vi "Write_Ch_data_file.vi"(4 "Append last row only":bool, 5 "Header string":string, 7 "exists?":bool, 8 "Write offset fr file end":i32, 9 "Channel Values":string[][](array[string]), 10 "Channel names":string[](array[string]), 11 "Filename":path) -> ()   [LabVIEW 2015]
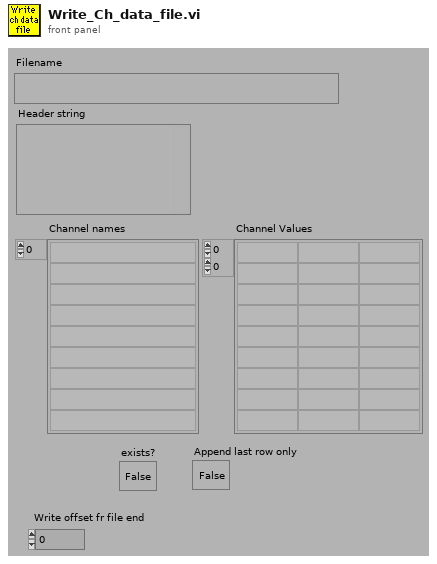
[diagram p1: front panel]
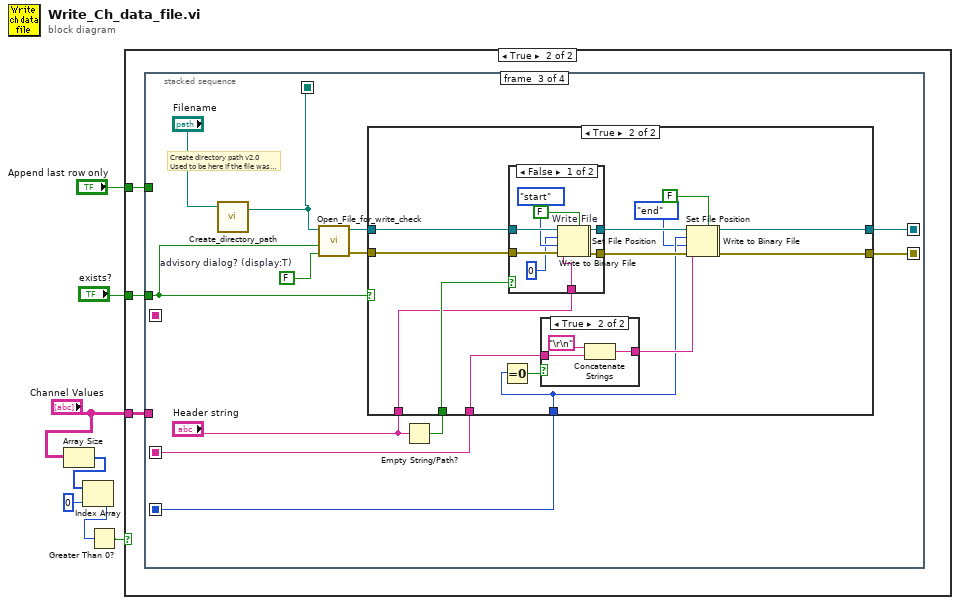
[diagram p0: block diagram]
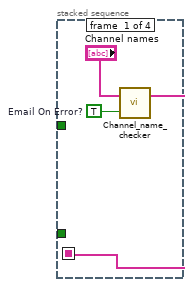
[diagram p3: hidden frame]
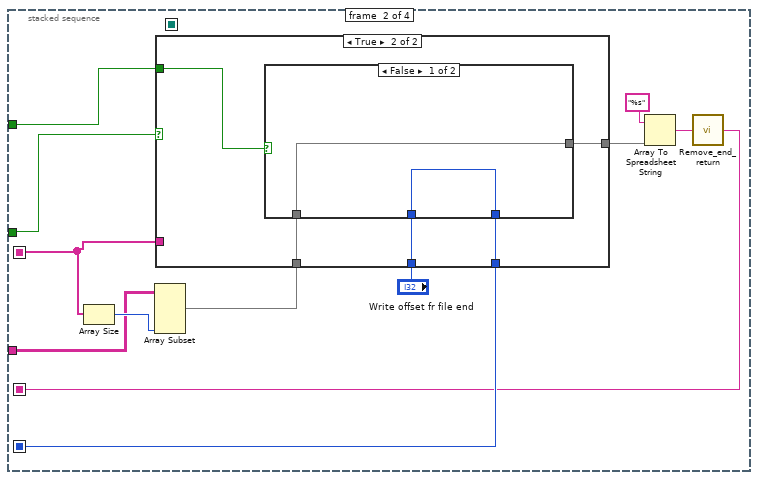
[diagram p4: hidden frame]
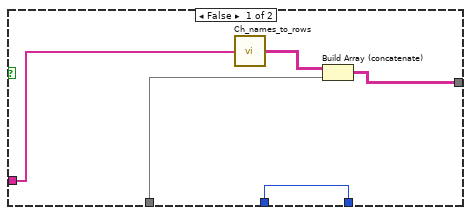
[diagram p5: hidden frame]
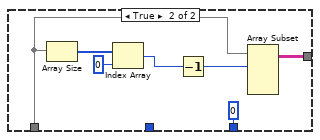
[diagram p6: hidden frame]
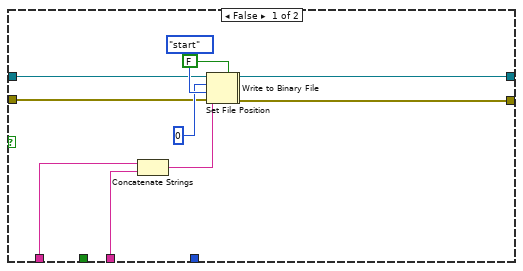
[diagram p7: hidden frame]
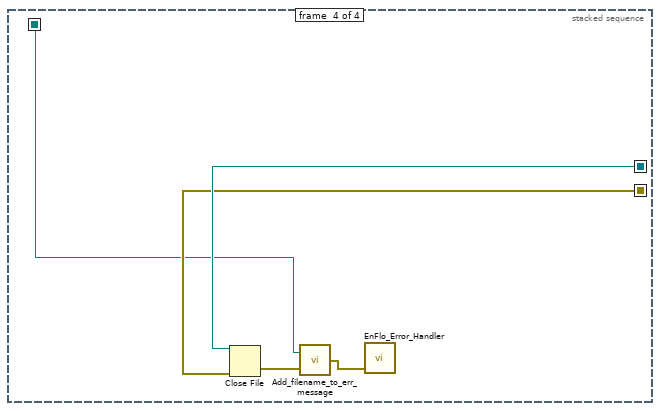
[diagram p10: hidden frame]
diagram:
  n1 = Array Size(array="Channel Values") -> (size(s)=w3:i32[])
  n2 = Index Array(array=w3, index=0 ("Index")) -> (element=w2:i32)
  n3 = Greater Than 0?(x=w2) -> (x > 0?=w1:bool)
  n4 = case shown="True" w1 {
    tunnel: "exists?" -> [_ w10]
    tunnel: "Append last row only" -> [_ w9]
    tunnel: "Channel Values" -> [_ w8]
    frame False {
    }
    frame True {
      n5 = stacked-sequence {
        seq-local: [_ w19 _ _] -> [_ _ w55 _]
        seq-local: [_ w22 _ _] -> [_ _ w52 _]
        seq-local: [_ _ w53 _] -> [_ _ _ w105]
        seq-local: [_ _ w51 _] -> [_ _ _ w104]
        seq-local: [w13 _ _ _] -> [_ w15 _ _]
        seq-local: [_ _ w45 _] -> [_ _ _ w102]
        tunnel: w10 -> [_ w21 w47 _]
        tunnel: w9 -> [_ w23 _ _]
        tunnel: w8 -> [_ w16 _ _]
        frame #0 {
          w11 = TRUE  # Email On Error?
          n6 = call "Channel_name_checker.vi"("Email On Error?"=w11, "Channel names"="Channel names") -> ("Channel names Out"=w13:string[])  [unwired: 1 out]
        }
        frame #1 {
          n7 = Array Size(array=w15) -> (size(s)=w17:i32)
          n8 = Array Subset(array=w16, length (col)=w17) -> (w14:string[][])  [unwired: 3 in]
          n9 = case shown="True" w21 {
            tunnel: w15 -> [w27 _]
            tunnel: [w30 w32] -> w24
            tunnel: w23 -> [_ w35]
            tunnel: [w29 w34] -> w22
            tunnel: "Write offset fr file end" -> [w29 w33]
            tunnel: w14 -> [w26 w31]
            frame False {
              n10 = call "Ch_names_to_rows.vi"("Channel Names"=w27) -> ("3 Row names"=w28:string[][])
              n11 = Build Array (concatenate)(w28, w26) -> (w30:string[][])
            }
            frame True {
              n12 = case shown="False" w35 {
                tunnel: w31 -> [w37 w40]
                tunnel: [w37 w39] -> w32
                tunnel: [w36 0 ("Write offset fr file end")] -> w34
                tunnel: w33 -> [w36 _]
                frame False {
                }
                frame True {
                  n13 = Array Size(array=w40) -> (size(s)=w43:i32[])
                  n14 = Index Array(array=w43, index=0) -> (element=w41:i32)
                  n15 = Decrement(x=w41) -> (x-1=w42:i32)
                  n16 = Array Subset(array=w40, index (row)=w42) -> (w39:string[][])  [unwired: 3 in]
                }
              }
            }
          }
          n17 = Array To Spreadsheet String(array=w24, 3:"%s" ("format string")) -> (spreadsheet string=w20:string)  [unwired: 1 out]
          n18 = call "Remove_end_return.vi"("Input string"=w20) -> ("Output string"=w19:string)
        }
        frame #2 {
          w49 = FALSE  # advisory dialog? (display:T)
          # "Create directory path v2.0\nUsed to be here if the file was new"
          n19 = call "Create_directory_path.vi"("Path name"="Filename") -> ("Path name Out"=w45:path)  [unwired: 2 in, 1 out]
          n20 = call "Open_File_for_write_check.vi"("advisory dialog? (display:T)"=w49, "append to file? (new file:F)"=w47, "file path"=w45) -> ("error out"=w50:errorcluster, "refnum"=w48:refnum<file>)  [unwired: 7 out]
          n21 = Empty String/Path?(string/path="Header string") -> (empty?=w56:bool)
          n22 = case shown="True" w47 {
            tunnel: w56 -> [_ w82]
            tunnel: w52 -> [_ w75]
            tunnel: w55 -> [w64 w78]
            tunnel: [w66 w81] -> w51
            tunnel: "Header string" -> [w65 w80]
            tunnel: [w62 w79] -> w53
            tunnel: w48 -> [w61 w73]
            tunnel: w50 -> [w60 w74]
            frame False {
              n23 = Concatenate Strings(w65, w64) -> (w63:string)
              n24 = Set File Position(offset (in bytes) (0)=0 ("pos offset (0)"), refnum=w61, from (0:start)=enum16{"start", "end", "current"}."start" ("pos mode (0:2)"), error in=w60) -> (refnum out=w59:refnum<file>, error out=w58:errorcluster)
              n25 = Write to Binary File(file (use dialog)=w59, data=w63, error in=w58, 5:FALSE ("prepend array or string size? (T)")) -> (refnum out=w62:refnum<file>, error out=w66:errorcluster)  [unwired: 3 out]
            }
            frame True {
              n26 = Equal To 0?(x=w75) -> (x = 0?=w76:bool)
              n27 = case shown="False" w82 {
                tunnel: w73 -> [w98 w100]
                tunnel: w74 -> [w97 w99]
                tunnel: [w94 w100] -> w84
                tunnel: [w93 w99] -> w83
                tunnel: w80 -> [w92 _]
                frame False {
                  n28 = Set File Position(offset (in bytes) (0)=0 ("pos offset (0)"), refnum=w98, from (0:start)=enum16{"start", "end", "current"}."start" ("pos mode (0:2)"), error in=w97) -> (refnum out=w91:refnum<file>, error out=w90:errorcluster)
                  n29 = Write to Binary File "Write File"(file (use dialog)=w91, data=w92, error in=w90, 5:FALSE ("prepend array or string size? (T)")) -> (refnum out=w94:refnum<file>, error out=w93:errorcluster)  [unwired: 3 out]
                }
                frame True {
                }
              }
              n30 = case shown="True" w76 {
                tunnel: w78 -> [w85 w88]
                tunnel: [w85 w87] -> w77
                frame False {
                }
                frame True {
                  n31 = Concatenate Strings("\r\n", w88) -> (w87:string)
                }
              }
              n32 = Set File Position(offset (in bytes) (0)=w75, refnum=w84, from (0:start)=enum16{"start", "end", "current"}."end" ("pos mode (0:2)"), error in=w83) -> (refnum out=w71:refnum<file>, error out=w70:errorcluster)
              n33 = Write to Binary File(file (use dialog)=w71, data=w77, error in=w70, 5:FALSE ("prepend array or string size? (T)")) -> (refnum out=w79:refnum<file>, error out=w81:errorcluster)  [unwired: 3 out]
            }
          }
        }
        frame #3 {
          n34 = Close File(refnum=w105, error in=w104) -> (error out=w103:errorcluster)  [unwired: 1 out]
          n35 = call "Add_filename_to_err_message.vi"("error in (no error)"=w103, "Path"=w102) -> ("error out"=w101:errorcluster)
          n36 = call "EnFlo_Error_Handler.vi"("error in (no error)"=w101) -> ()  [unwired: 2 in, 3 out]
        }
      }
    }
  }
